vi "find_nearest.vi"(9 "Sorted Array (<)":dbl[](array[numeric]), 10 "Key":dbl) -> (0 "Lower":dbl, 1 "Nearest index":i32, 2 "Nearest":dbl, 3 "Upper":dbl)   [LabVIEW 2019]
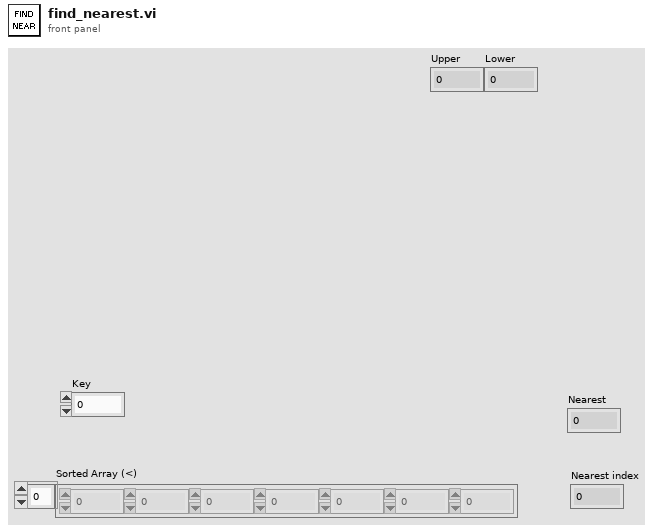
[diagram p1: front panel]
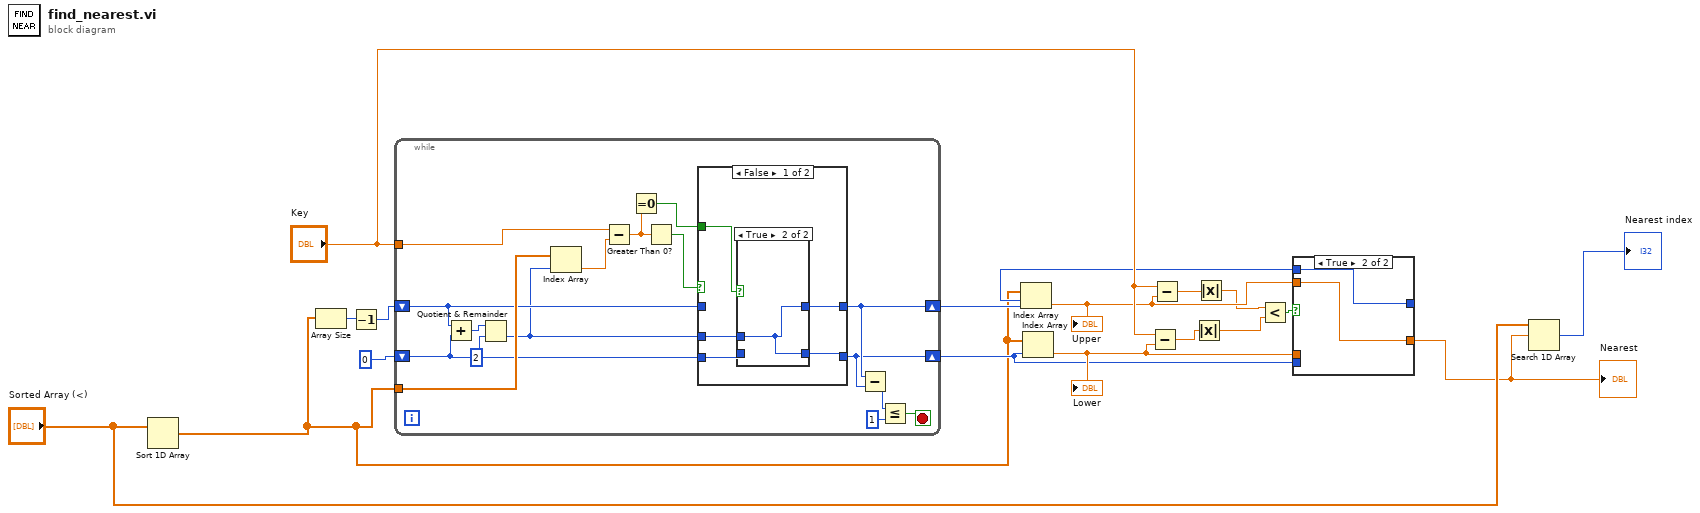
[diagram p0: block diagram]
diagram:
  n1 = Sort 1D Array(array="Sorted Array (<)") -> (sorted array=w4:dbl[])
  n2 = Array Size(array=w4) -> (size(s)=w17:i32)
  n3 = Decrement(x=w17) -> (x-1=w16:i32)
  n4 = while {
    shift-right: [w22] -> w10
    shift-left: w16 -> [w28]
    shift-right: [w21] -> w9
    shift-left: 0 -> [w27]
    tunnel: w4 -> [w31]
    tunnel: "Key" -> [w30]
    stop <- w18 stop-if-true
    n5 = Add(x=w28, y=w27) -> (x+y=w33:i32)
    n6 = Quotient & Remainder(x=w33, y=2) -> (floor(x/y)=w25:i32)  [unwired: 1 out]
    n7 = Index Array(array=w31, index=w25) -> (element=w29:dbl)
    n8 = Subtract(x=w30, y=w29) -> (x-y=w24:dbl)
    n9 = Equal To 0?(x=w24) -> (x = 0?=w23:bool)
    n10 = Greater Than 0?(x=w24) -> (x > 0?=w26:bool)
    n11 = case shown="False" w26 {
      tunnel: w28 -> [_ w42]
      tunnel: w27 -> [w35 _]
      tunnel: w25 -> [w36 w43]
      tunnel: [w34 w43] -> w21
      tunnel: [w37 w42] -> w22
      tunnel: w23 -> [w38 _]
      frame False {
        n12 = case shown="True" w38 {
          tunnel: [w40 w41] -> w37
          tunnel: w36 -> [w40 w41]
          tunnel: w35 -> [w39 _]
          tunnel: [w39 w41] -> w34
          frame False {
          }
          frame True {
          }
        }
      }
      frame True {
      }
    }
    n13 = Subtract(x=w22, y=w21) -> (x-y=w20:i32)
    n14 = Less Or Equal?(x=w20, y=1) -> (x <= y?=w18:bool)
  }
  n15 = Index Array(array=w4, index=w10) -> (element=w12:dbl)
  "Upper" <- w12
  n16 = Index Array(array=w4, index=w9) -> (element=w11:dbl)
  "Lower" <- w11
  n17 = Subtract(x="Key", y=w11) -> (x-y=w6:dbl)
  n18 = Subtract(x="Key", y=w12) -> (x-y=w8:dbl)
  n19 = Absolute Value(x=w6) -> (abs(x)=w5:dbl)
  n20 = Absolute Value(x=w8) -> (abs(x)=w7:dbl)
  n21 = Less?(x=w7, y=w5) -> (x < y?=w13:bool)
  n22 = case shown="True" w13 {
    tunnel: w10 -> [_ w47]
    tunnel: [w44 w47] -> _
    tunnel: w12 -> [_ w46]
    tunnel: [w45 w46] -> w2
    tunnel: w9 -> [w44 _]
    tunnel: w11 -> [w45 _]
    frame False {
    }
    frame True {
    }
  }
  "Nearest" <- w2
  n23 = Search 1D Array(1D array="Sorted Array (<)", element=w2) -> (index of element=→"Nearest index":i32)  [unwired: 1 in]
